vi "ZeroVector.vi"() -> (0 "Zero Vector":refnum<class "Vector2.lvclass">)   [LabVIEW 2022 SP3, in "Vector2.lvclass"]
uses:
  Vector2.lvclass
  Vector2.lvclass/Vector2.ctl
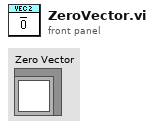
[diagram p1: front panel]
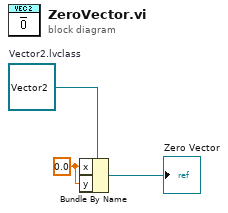
[diagram p0: block diagram]
diagram:
  w1 = sgl 0.0 ("x")
  w2 = refnum<class "Vector2.lvclass"> refnum  # Vector2.lvclass
  n1 = Bundle By Name(cluster=w2, "x"=w1, "y"=w1) -> (→"Zero Vector":refnum<class "Vector2.lvclass">)
